vi "Set Setpoint.vi"(8 "error in":errorcluster, 9 "Data":variant, 10 "Ident":string, 11 "Task Actor in":refnum<class "Task Actor.lvclass">) -> (0 "error out":errorcluster, 3 "Task Actor out":refnum<class "Task Actor.lvclass">)   [LabVIEW 2024, in "Task Actor.lvlib" / "Task Actor.lvclass"]
uses:
  Task Actor.lvclass
  Task Actor.lvclass/Task Actor.ctl
  <vilib>/Utility/miscctls.llb/LVMapReplaceAction.ctl
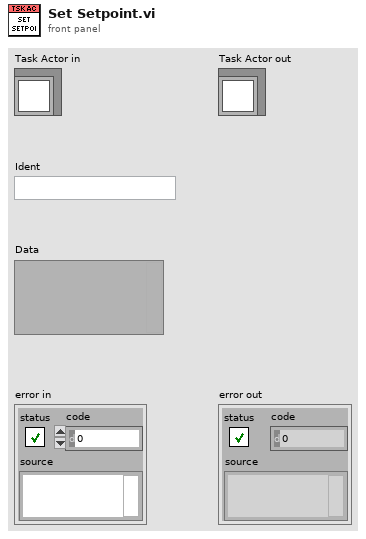
[diagram p1: front panel]
types:
  T1 = typedef "LVMapReplaceAction.ctl" = enum32{"Modify Entry only if found", "Add or Modify Entry", "Delete Entry"}
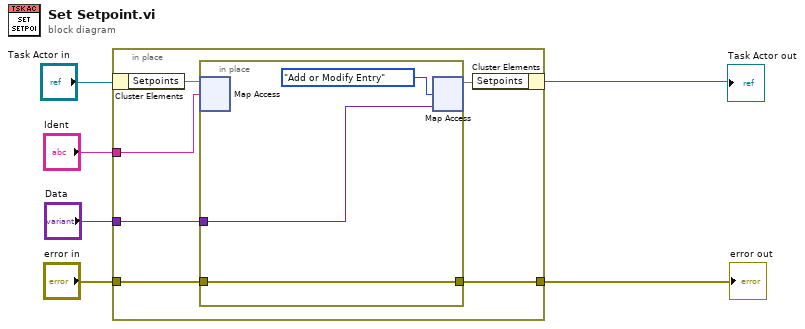
[diagram p0: block diagram]
diagram:
  n1 = in-place {
    in-place-border: "Ident" -> [w11]
    in-place-border: "Data" -> [w10]
    in-place-border: "error in" -> [w8]
    in-place-border: [w7] -> w1
    n2 = in-place-cluster #1("Task Actor in") -> ("Setpoints"=w12:map{string, variant})
    n3 = in-place {
      in-place-border: w10 -> [w14]
      in-place-border: w8 -> [w13]
      in-place-border: [w13] -> w7
      n4 = in-place-map #2(w12, w11) -> ()  [unwired: 1 in, 2 out]
      n5 = in-place-map #2(w14, LVMapReplaceAction."Add or Modify Entry" ("action")) -> (w9:map{string, variant})  [unwired: 2 out]
    }
    n6 = in-place-cluster #1("Setpoints"=w9) -> (→"Task Actor out":refnum<class "Task Actor.lvclass">)
  }
  "error out" <- w1
